vi "teste 2.vi"() -> ()   [LabVIEW 2021]
uses:
  <vilib>/numeric/Random Number (Range) DBL.vi
  <vilib>/Analysis/3filter.llb/Butterworth Filter (DBL).vi
  <vilib>/Utility/file.llb/Write Delimited Spreadsheet (DBL).vi
  <vilib>/measure/NI_MABase.lvlib
  <vilib>/Analysis/NI_AALBase.lvlib
  <vilib>/ptbypt/NI_PtbyPt.lvlib
panel:
  in  "intervals":i32=10
  out "XY Graph":T1(graph)
  in  "high cutoff freq: fh":dbl=0.45000000000000007 format="%0.2f"
  out "Waveform Graph 4":dbl[](graph)
  out "Numeric":dbl
  out "Waveform Graph 3":dbl[](graph)
  out "Waveform Graph 2":dbl[](graph)
  out "Waveform Graph":dbl[](graph)
  out "x*y":dbl
  out "number":dbl
  in  "stop":bool
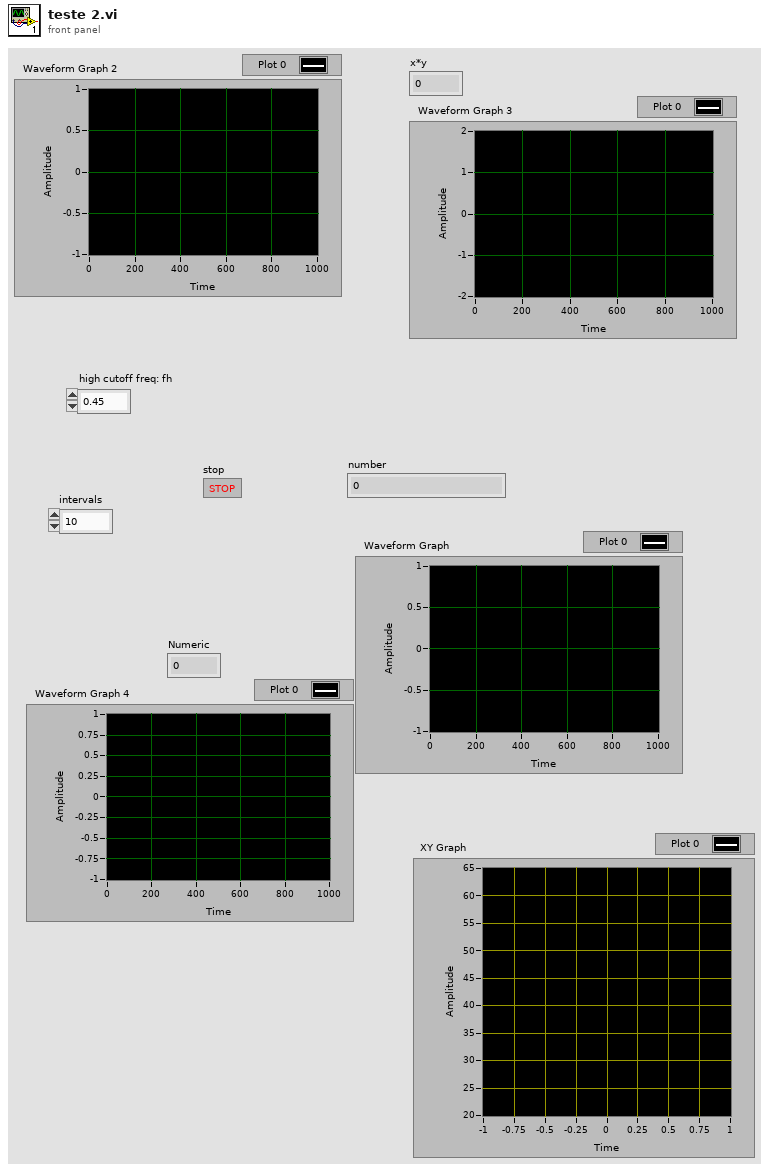
[diagram p1: front panel]
types:
  T1 = cluster{"X Values":dbl[], "Histogram: h(x)":i32[]}
  T2 = enum16{"open", "replace", "create", "open or create", "replace or create", "replace or create with confirmation"}
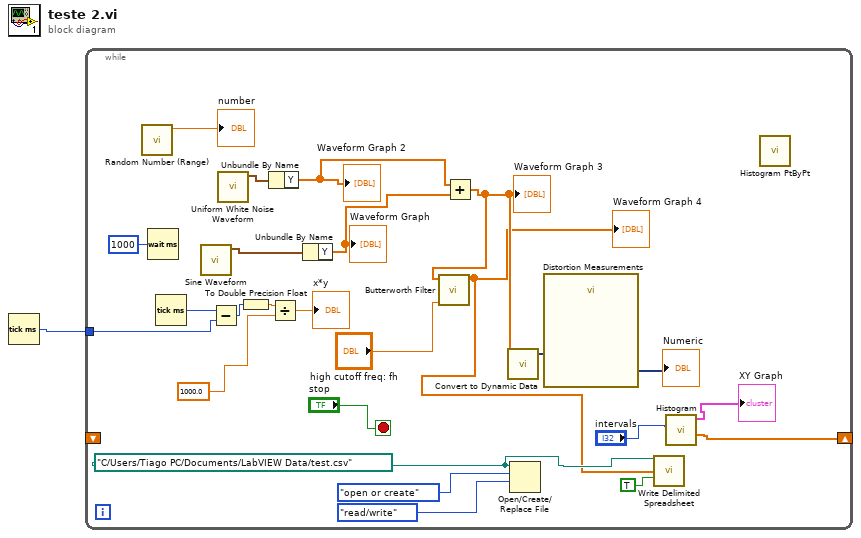
[diagram p0: block diagram]
diagram:
  n1 = Tick Count (ms)() -> (millisecond timer value=w1:u32)
  n2 = while {
    tunnel: w1 -> [w23]
    shift-right: [w5] -> _
    shift-left: _ -> [_]
    stop <- "stop" stop-if-true
    w8 = path "C:/Users/Tiago PC/Documents/LabVIEW Data/test.csv" ("Filename")
    n3 = call-poly <vilib>:"Random Number (Range).vi"() -> ("number"=→"number":dbl)  [unwired: 11 in]
    n4 = Wait (ms)(milliseconds to wait=u32 1000) -> ()  [unwired: 1 out]
    n5 = Tick Count (ms)() -> (millisecond timer value=w24:u32)
    n6 = call <vilib>:"Sine Waveform.vi"() -> ("signal out"=w20:waveform(dbl))  [unwired: 10 in, 1 out]
    n7 = Subtract(x=w24, y=w23) -> (x-y=w21:u32)
    n8 = call <vilib>:"Uniform White Noise Waveform.vi"() -> ("signal out"=w18:waveform(dbl))  [unwired: 10 in, 1 out]
    n9 = To Double Precision Float(number=w21) -> (double precision float=w12:dbl)
    n10 = Unbundle By Name(w18) -> ("Y"=w17:dbl[])
    "Waveform Graph 2" <- w17
    n11 = Divide(x=w12, y=1000.0 ("x")) -> (x/y=→"x*y":dbl)
    n12 = Unbundle By Name(w20) -> ("Y"=w16:dbl[])
    "Waveform Graph" <- w16
    n13 = Add(x=w17, y=w16) -> (x+y=w11:dbl[])
    "Waveform Graph 3" <- w11
    n14 = call-poly <vilib>:"Butterworth Filter.vi"("low cutoff freq: fl"="high cutoff freq: fh", "X"=w11) -> ("Filtered X"=w3:dbl[])  [unwired: 6 in, 1 out]
    "Waveform Graph 4" <- w3
    n15 = call "Convert to Dynamic Data"("Array"=w11) -> ("Dynamic Data Type"=w15:dynamicdata)  [unwired: 3 in]
    n16 = Open/Create/Replace File(file path (use dialog)=w8, operation (0:open)=T2."open or create", access (0:read/write)=enum16{"read/write", "read-only", "write-only"}."read/write") -> ()  [unwired: 3 in, 3 out]
    n17 = call "Distortion Measurements"("Signals"=w15) -> ("SINAD (dB)"=→"Numeric":dynamicdata)  [unwired: 9 in, 1 out]
    n18 = call-poly <vilib>:"Write Delimited Spreadsheet.vi"("file path (dialog if empty)"=w8, "1D data"=w3, "append to file? (new file:F)"=TRUE) -> ()  [unwired: 11 in, 2 out]
    n19 = call <vilib>:"Histogram.vi"("intervals"="intervals") -> ("X Values"=w5:dbl[], "Histogram Graph"=→"XY Graph":T1)  [unwired: 7 in, 2 out]
    n20 = call <vilib>:"Histogram PtByPt.vi"() -> ()  [unwired: 8 in, 4 out]
  }
